vi "NKT_Init.vi"(8 "entrée d'erreur (pas d'erreur)":errorcluster) -> (0 "sortie d'erreur":errorcluster, 2 "portname":string, 3 "Found?":bool)   [LabVIEW 2026]
uses:
  Controls/TypeDef_FGV.ctl
  <instrlib>/NKTP_API/NKTP_API.lvlib
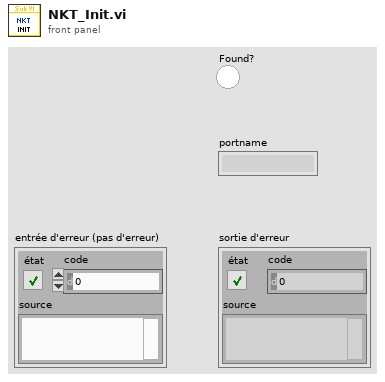
[diagram p1: front panel]
types:
  T1 = typedef "TypeDef_FGV.ctl" = enum16{"Initialize", "Write", "Read"}
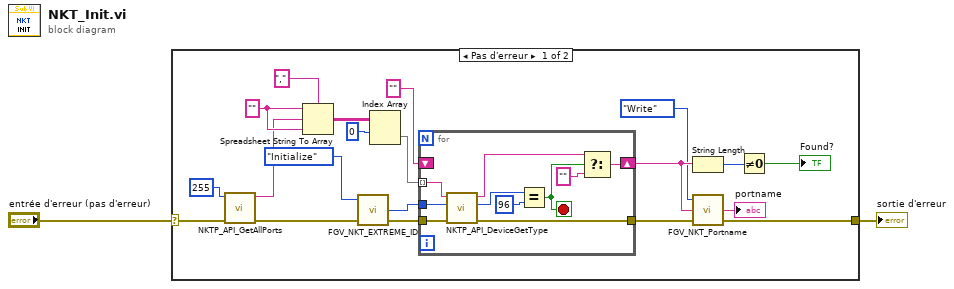
[diagram p0: block diagram]
diagram:
  n1 = case shown="Pas d'erreur" "entrée d'erreur (pas d'erreur)" {
    selector: "entrée d'erreur (pas d'erreur)" -> [w12 w33]
    tunnel: [w4 w33] -> w2
    frame No Error {
      w16 = ""
      n2 = call <instrlib>:"NKTP_API_GetAllPorts.vi"("error in"=w12, "maxLen"=u16 255) -> ("error out"=w10:errorcluster, "portnames"=w14:string)  [unwired: 8 in]
      n3 = Spreadsheet String To Array(delimiter (Tab)="," ("séparateur (Tabulation)"), format string=w16, spreadsheet string=w14, array type (2D Dbl)=w16) -> (array=w18:string[][])
      n4 = call "FGV_NKT_EXTREME_ID.vi"("error in"=w10, "Action"=TypeDef_FGV."Initialize") -> ("error out"=w9:errorcluster, "ID"=w8:i32)  [unwired: 2 in]
      n5 = Index Array(array=w18, index (row)=0 ("indice (ligne)")) -> (element=w19:string[])  [unwired: 1 in]
      n6 = for {
        tunnel: [w32] -> w5
        tunnel: w9 -> [w31]
        tunnel: w19 -> [w30] mode=indexing
        shift-right: [w25] -> w7
        shift-left: "" ("portname") -> [_]
        tunnel: w8 -> [w23]
        stop <- w27 stop-if-true
        n7 = call <instrlib>:"NKTP_API_DeviceGetType.vi"("error in"=w31, "devId"=w23, "portname"=w30) -> ("error out"=w32:errorcluster, "devType"=w29:u8, "portname"=w26:string)  [unwired: 6 in]
        n8 = Equal?(x=w29, y=u8 96) -> (x = y?=w27:bool)
        n9 = Select(t=w26, s=w27, f="" ("cas faux")) -> (s? t:f=w25:string)
      }
      n10 = String Length(string=w7) -> (length=w22:i32)
      n11 = call "FGV_NKT_Portname.vi"("error in"=w5, "Portname"=w7, "Action"=TypeDef_FGV."Write") -> ("error out"=w4:errorcluster, "Portname"=→"portname":string)  [unwired: 1 in]
      n12 = Not Equal To 0?(x=w22) -> (x != 0?=→"Found?":bool)
    }
    frame Error {
    }
  }
  "sortie d'erreur" <- w2
